vi "解析xml.vi"() -> ()   [LabVIEW 2017]
uses:
  <vilib>/xml/Load XML File.vi
  <vilib>/xml/NI_XML.lvlib
  <resource>/objmgr/DOMUserDefRef.rc
panel:
  out "XML Elements":string[](array[string]) caption="XML元素"
  out "Xml字符串":string
  out "实验0001":T1
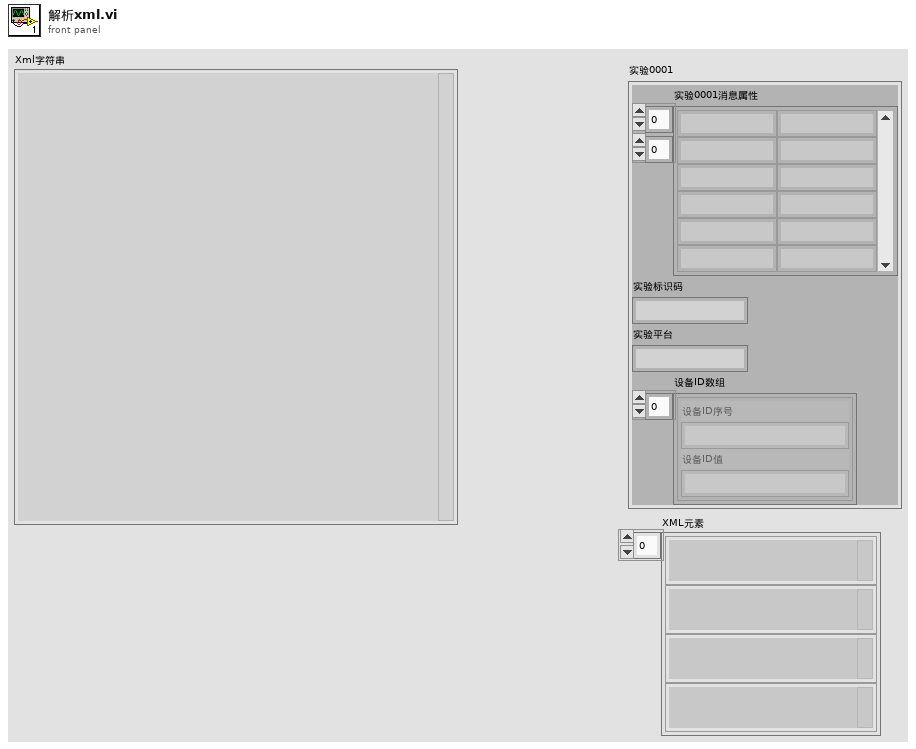
[diagram p1: front panel]
types:
  T1 = cluster{"实验0001消息属性":string[][], "实验标识码":string, "实验平台":string, "设备ID数组":cluster{"设备ID序号":string, "设备ID值":string}[]}
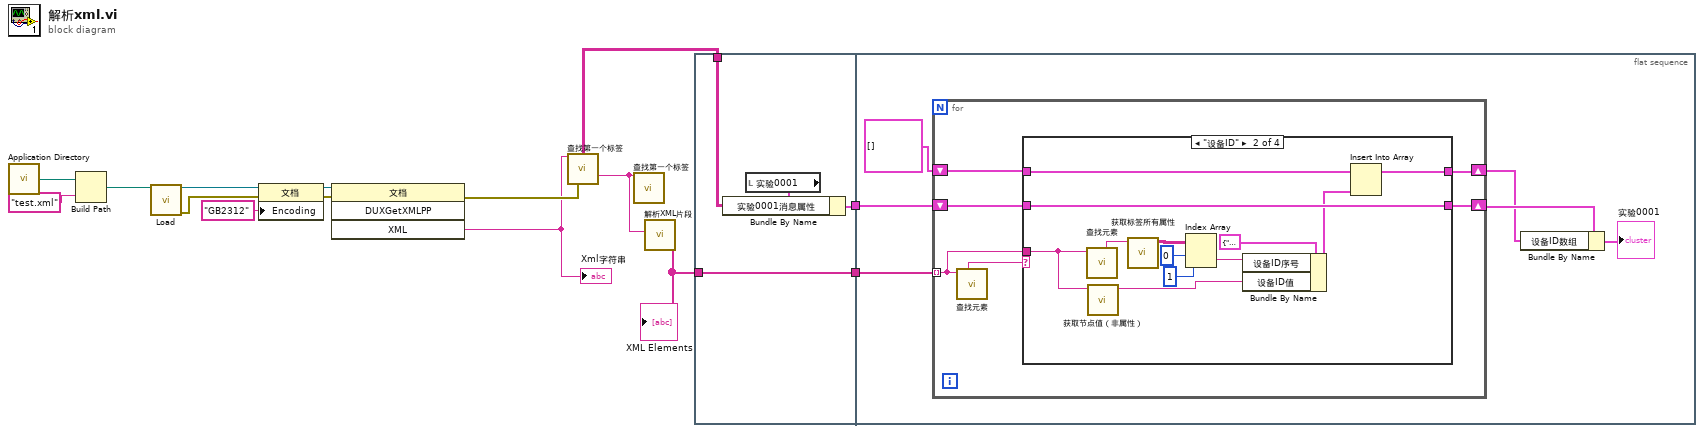
[diagram p0: block diagram]
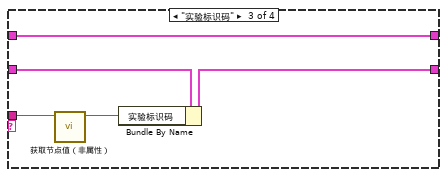
[diagram p3: hidden frame]
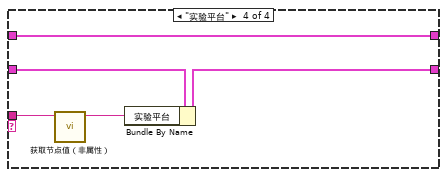
[diagram p4: hidden frame]
diagram:
  n1 = call <vilib>:"Application Directory.vi"() -> ("Application Directory"=w15:path)
  n2 = Build Path(base path=w15, name or relative path="test.xml" ("名称或相对路径")) -> (appended path=w14:path)
  n3 = call-poly <vilib>:"Load.vi"("path to XML document"=w14) -> ("DOM document out"=w12:refnum<k20>, "error out"=w10:errorcluster)  [unwired: 12 in, 1 out]
  n4 = property class="文档"(reference=w12, error in=w10, "Encoding"="GB2312" ("文档编码")) -> (reference out=w9:refnum<k20>, error out=w8:errorcluster)
  n5 = invoke class="文档" method="DUXGetXMLPP"(reference=w9, error in=w8) -> (error out=w7:errorcluster, "XML"=w6:string)  [unwired: 2 in, 2 out]
  "Xml字符串" <- w6
  n6 = call "查找第一个标签.vi"("XML String In"=w6, "error in (no error)"=w7) -> ("xml node attribute out"=w2:string[][], "after tag"=w5:string)  [unwired: 5 in, 7 out]
  n7 = call "查找第一个标签.vi"("XML String In"=w5) -> ()  [unwired: 6 in, 9 out]
  n8 = call "解析XML片段.vi"("XML in"=w5) -> ("XML Elements"=w4:string[])  [unwired: 9 in, 1 out]
  "XML Elements" <- w4
  n9 = flat-sequence {
    tunnel: w4 -> [w19]
    tunnel: [w19] -> w3
    tunnel: w2 -> [w18]
    tunnel: [w16] -> w1
    tunnel: w3 -> [w25]
    tunnel: w1 -> [w24]
    frame #0 {
      n10 = local read "实验0001"() -> (w17:T1)
      n11 = Bundle By Name(cluster=w17, "实验0001消息属性"=w18) -> (w16:T1)
    }
    frame #1 {
      n12 = for {
        tunnel: w25 -> [w30] mode=indexing
        shift-right: [w28] -> w21
        shift-left: cluster{"航线ID序号":string, "航线ID值":string}[] [] ("航线ID数组") -> [w27]
        shift-right: [w26] -> w22
        shift-left: w24 -> [w29]
        n13 = call "查找元素.vi"("XML String In"=w30) -> ("节点名"=w31:string)  [unwired: 4 in, 6 out]
        n14 = case shown="\"设备ID\"" w31 {
          tunnel: w30 -> [_ w43 w50 w55]
          tunnel: w29 -> [w32 w37 w49 w54]
          tunnel: w27 -> [w33 w44 w47 w52]
          tunnel: [w33 w38 w47 w52] -> w28
          tunnel: [w32 w37 w46 w51] -> w26
          frame "假", Default {
          }
          frame "设备ID" {
            n15 = call "查找元素.vi"("XML String In"=w43) -> ("element name"=w45:string)  [unwired: 4 in, 6 out]
            n16 = call "获取节点值（非属性）.vi"("Xml Node"=w43) -> ("Xml Node Value"=w42:string)  [unwired: 10 in]
            n17 = call "获取标签所有属性.vi"("XML Node String In"=w45) -> ("xml attribute out"=w41:string[][])  [unwired: 8 in, 2 out]
            n18 = Index Array(array=w41, index (row)=0 ("索引 (行)"), index (col)=1 ("禁用的索引 (列)")) -> (element=w36:string)
            n19 = Bundle By Name(cluster=cluster{"设备ID序号":string, "设备ID值":string} {"设备ID序号"="", "设备ID值"=""} ("航线ID"), "设备ID序号"=w36, "设备ID值"=w42) -> (w34:cluster{"设备ID序号":string, "设备ID值":string})
            n20 = Insert Into Array(array=w44, new element=w34) -> (w38:cluster{"航线ID序号":string, "航线ID值":string}[])  [unwired: 1 in]
          }
          frame "实验标识码" {
            n21 = call "获取节点值（非属性）.vi"("Xml Node"=w50) -> ("Xml Node Value"=w48:string)  [unwired: 10 in]
            n22 = Bundle By Name(cluster=w49, "实验标识码"=w48) -> (w46:T1)
          }
          frame "实验平台" {
            n23 = call "获取节点值（非属性）.vi"("Xml Node"=w55) -> ("Xml Node Value"=w53:string)  [unwired: 10 in]
            n24 = Bundle By Name(cluster=w54, "实验平台"=w53) -> (w51:T1)
          }
        }
      }
      n25 = Bundle By Name(cluster=w22, "设备ID数组"=w21) -> (→"实验0001":T1)
    }
  }
